vi "CamCalibration (SubVI).vi"(8 "error in":errorcluster, 10 "Image Dst":T2, 11 "Image In":T2) -> (0 "error out":errorcluster, 3 "Image Out":T2)   [LabVIEW 2019]
uses:
  <vilib>/vision/Image Controls.llb/IMAQ Image.ctl
  <vilib>/vision/NI_Vision_Development_Module.lvlib
panel:
  out "視覺參數read":T1
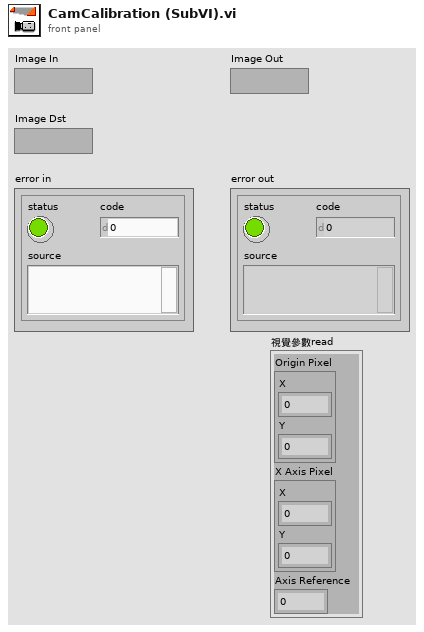
[diagram p1: front panel]
types:
  T1 = cluster{"Origin Pixel":cluster{"X":sgl, "Y":sgl}, "X Axis Pixel":cluster{"X":sgl, "Y":sgl}, "Axis Reference":u32}
  T2 = typedef "IMAQ Image.ctl" = refnum<image>
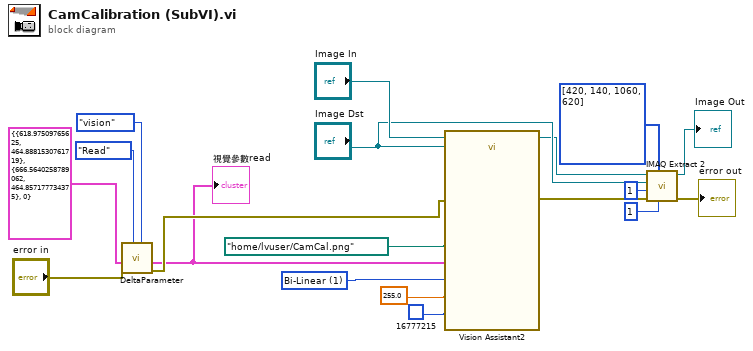
[diagram p0: block diagram]
diagram:
  w15 = u32 1 items=["Zero Order", "Bi-Linear", "Quadratic", "Cubic Spline"] ("Interpolation Type (Image Correction 1)")
  n1 = call "DeltaParameter.vi"("parameter"=enum16{"angle", "robot", "vision"}."vision", "mode"=enum16{"Read", "Write"}."Read", "error in (no error)"="error in", "視覺參數write"=T1 {"Origin Pixel"={"X"=618.9751, "Y"=464.88815}, "X Axis Pixel"={"X"=666.564, "Y"=464.85718}, "Axis Reference"=0} ("Calibration Axis Info (Image Calibration 1)")) -> ("error out"=w11:errorcluster, "視覺參數read"=w9:T1)  [unwired: 3 in, 3 out]
  "視覺參數read" <- w9
  n2 = call "Vision Assistant2"("Image In"="Image In", "Image Dst"="Image Dst", "Calibration Axis Info (Image Calibration 1)"=w9, "Interpolation Type (Image Correction 1)"=w15, "Replace Value (Image Correction 1)"=sgl 255.0, "Color Replace Value (Image Correction 1)"=u32 16777215, "File Path (Image Calibration 1)"=path "/home/lvuser/CamCal.png", "error in"=w11) -> ("Image Out"=w5:T2, "error out"=w8:errorcluster)  [unwired: 18 in]
  n3 = call "IMAQ Extract 2"("Y Step Size"=1, "Optional Rectangle"=i32[] [420, 140, 1060, 620], "error in (no error)"=w8, "X Step Size"=1, "Image Dst"="Image Dst", "Image Src"=w5) -> ("error out"=→"error out":errorcluster, "Image Dst Out"=→"Image Out":T2)  [unwired: 4 in]
